vi "Modify Item.vi"(6 "Data":variant, 8 "error in (no error)":errorcluster, 9 "Text":string, 10 "Tag":refnum<class "Tree Tag Class.lvclass">, 11 "Tree_LVOOP in":refnum<class "Tree Class.lvclass">) -> (0 "error out":errorcluster, 2 "Tag dup":refnum<class "Tree Tag Class.lvclass">, 3 "Tree_LVOOP out":refnum<class "Tree Class.lvclass">)   [LabVIEW 2012, in "Tree Tools.lvlib" / "Tree Class.lvclass"]
uses:
  Tree Class.lvclass
  Tree Tag Class/Tree Tag Class.lvclass
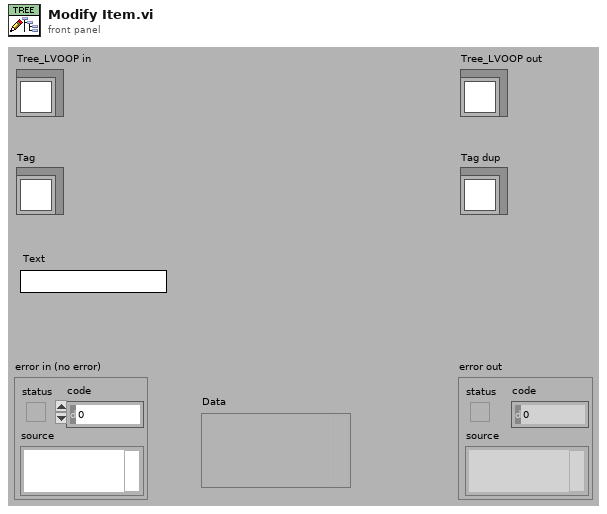
[diagram p1: front panel]
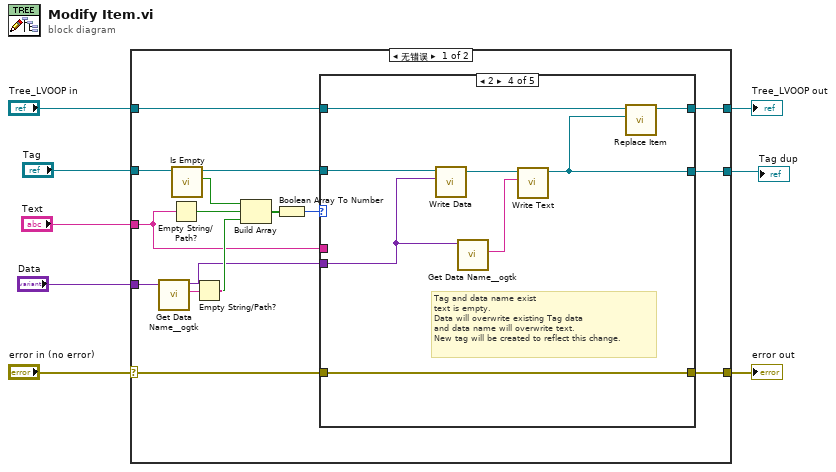
[diagram p0: block diagram]
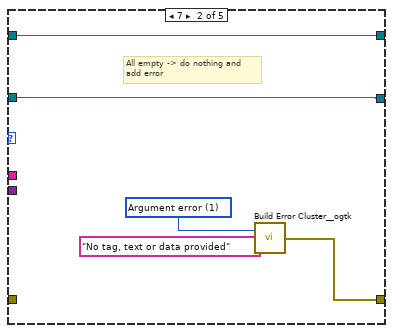
[diagram p3: hidden frame]
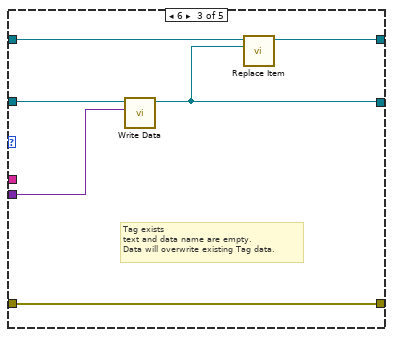
[diagram p4: hidden frame]
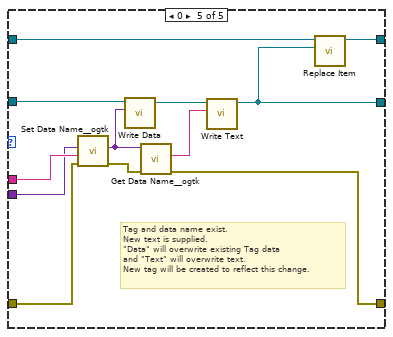
[diagram p5: hidden frame]
diagram:
  n1 = case shown="无错误" "error in (no error)" {
    selector: "error in (no error)" -> [w16 w61]
    tunnel: [w15 w61] -> w7
    tunnel: [w13 w60] -> w5
    tunnel: "Tree_LVOOP in" -> [w14 w60]
    tunnel: "Tag" -> [w24 w59]
    tunnel: "Text" -> [w11 _]
    tunnel: "Data" -> [w23 _]
    tunnel: [w9 w59] -> w1
    frame No Error {
      n2 = call <userlib>:"Get Data Name__ogtk.vi"("Data"=w23) -> ("Data Name"=w22:string, "Data dup"=w10:variant)  [unwired: 1 in, 8 out]
      n3 = Empty String/Path?(string/path=w11) -> (empty?=w20:bool)
      n4 = call-dynamic "Is Empty.vi"("Tag_LVOOP in"=w24) -> ("Empty"=w21:bool, "Tag_LVOOP out"=w12:refnum<class "Tree Tag Class.lvclass">)  [unwired: 8 in, 1 out]
      n5 = Empty String/Path?(string/path=w22) -> (empty?=w19:bool)
      n6 = Build Array(w21, w20, w19) -> (w18:bool[])
      n7 = Boolean Array To Number(Boolean array=w18) -> (number=w17:u32)
      n8 = case shown="2" w17 {
        tunnel: w16 -> [w26 _ w38 w46 w48]
        tunnel: [w26 w31 w38 w46 w47] -> w15
        tunnel: w14 -> [w27 w32 w35 w44 w57]
        tunnel: [w27 w32 w34 w43 w56] -> w13
        tunnel: w12 -> [w25 w28 w37 w45 w58]
        tunnel: w11 -> [_ _ _ _ w53]
        tunnel: w10 -> [_ _ w36 w41 w52]
        tunnel: [w25 w28 w33 w39 w54] -> w9
        frame Default {
        }
        frame 7 {
          w30 = 1 items=["No error", "Argument error", "Memory is full", "Out of zone", "End of file", "File already open", "Generic file I/O error", "File not found", "File permission error", "Disk is full", "Duplicate path", "Too many files open", "System feature not enabled", "Resource file not found", "Cannot add resource", "Resource not found", "Image not found", "Image memory error", "Pen does not exist", "Config type invalid", "Config token not found", "Config parse error", "Config memory error", "Bad external code format", "Bad external code offset", "External code not present", "Null window", "Destroy window error", "Null menu", "Print aborted", "Bad print record", "Print driver error", "Windows error during printing", "Memory error during printing", "Print dialog error", "Generic print error", "Invalid device refnum", "Device not found", "Device parameter error", "Device unit error", "Cannot open device", "Device call aborted", "Generic error", "Cancelled by user", "Object ID too low", "Object ID too high", "Object not in heap", "Unknown heap", "Unknown object (invalid DefProc)", "Unknown object (DefProc not in table)", "Message out of range", "Invalid (null) method", "Unknown message", "Manager call not supported", "Bad address", "Network operation in progress", "Network operation timed out", "Connection is busy", "Network attribute not supported", "Network error", "Address in use", "System out of memory", "Connection aborted", "Connection refused", "Not connected", "Already connected", "Connection closed", "Initialization error (interapplication manager)", "Bad occurrence", "Wait on unbound occurrence handler", "Occurrence queue overflow", "Datalog type conflict", "Unused", "Unrecognized type (interapplication manager)", "Memory corrupt", "Failed to make temporary DLL", "Old CIN version", "Drag socket not found", "Failed to load drop-object", "Failed to register OLE object", "Failed to release OLE object", "Format specifier type mismatch", "Unknown format specifier", "Too few format specifiers", "Too many format specifiers", "Scan failed", "Newer CIN version", "Error converting to variant", "Runtime menu error", "Password tampered", "Variant attribute not found", "Incompatible variant data type", "Event data is not available", "Event Store is not present", "Occurrence is not found", "Event Queue is not created", "Event info is not available", "Refnum passed is NULL", "Error retrieving Class GUID", "Error retrieving CoClass GUID", "Error retrieving TypeLib GUID.", "Bad built application magic bytes.", "Specific driver is different from the specific driver associated with the Logical Name.", "There is no session opened to the class driver.", "Max Error", "MAX - Error with config objects", "MAX - Error loading configuration", "MAX - Group not supported"]
          # "All empty -> do nothing and\nadd error"
          n9 = call <userlib>:"Build Error Cluster__ogtk.vi"("String to Prepend to source (\"\")"="No tag, text or data provided" ("String to Prepend to source (\"\")"), "code"=w30) -> ("error out"=w31:errorcluster)
        }
        frame 6 {
          # "Tag exists\ntext and data name are empty.\nData will overwrite existing Tag data."
          n10 = call-dynamic "Write Data.vi"("Data"=w36, "Tag_LVOOP.lvclass in"=w37) -> ("Tag_LVOOP.lvclass out"=w33:refnum<class "Tree Tag Class.lvclass">)  [unwired: 8 in, 1 out]
          n11 = call-dynamic "Replace Item.vi"("Tag"=w33, "Tree_LVOOP in"=w35) -> ("Tree_LVOOP out"=w34:refnum<class "Tree Class.lvclass">)  [unwired: 1 in, 8 out]
        }
        frame 2 {
          # "Tag and data name exist\ntext is empty.\nData will overwrite existing Tag data\nand data name will overwrite text.\nNew tag will be created to reflect this change."
          n12 = call-dynamic "Write Data.vi"("Data"=w41, "Tag_LVOOP.lvclass in"=w45) -> ("Tag_LVOOP.lvclass out"=w42:refnum<class "Tree Tag Class.lvclass">)  [unwired: 8 in, 1 out]
          n13 = call <userlib>:"Get Data Name__ogtk.vi"("Data"=w41) -> ("Data Name"=w40:string)  [unwired: 1 in, 9 out]
          n14 = call-dynamic "Write Text.vi"("Text"=w40, "Tag_LVOOP.lvclass in"=w42) -> ("Tag_LVOOP.lvclass out"=w39:refnum<class "Tree Tag Class.lvclass">)  [unwired: 8 in, 1 out]
          n15 = call-dynamic "Replace Item.vi"("Tag"=w39, "Tree_LVOOP in"=w44) -> ("Tree_LVOOP out"=w43:refnum<class "Tree Class.lvclass">)  [unwired: 1 in, 8 out]
        }
        frame 0 {
          # "Tag and data name exist.\nNew text is supplied.\n\"Data\" will overwrite existing Tag data\nand \"Text\" will overwrite text.\nNew tag will be created to reflect this change."
          n16 = call <userlib>:"Set Data Name__ogtk.vi"("error in (no error)"=w48, "Data Name"=w53, "Data"=w52) -> ("error out"=w49:errorcluster, "Renamed Data"=w51:variant)  [unwired: 7 out]
          n17 = call-dynamic "Write Data.vi"("Data"=w51, "Tag_LVOOP.lvclass in"=w58) -> ("Tag_LVOOP.lvclass out"=w55:refnum<class "Tree Tag Class.lvclass">)  [unwired: 8 in, 1 out]
          n18 = call <userlib>:"Get Data Name__ogtk.vi"("error in (no error)"=w49, "Data"=w51) -> ("error out"=w47:errorcluster, "Data Name"=w50:string)  [unwired: 8 out]
          n19 = call-dynamic "Write Text.vi"("Text"=w50, "Tag_LVOOP.lvclass in"=w55) -> ("Tag_LVOOP.lvclass out"=w54:refnum<class "Tree Tag Class.lvclass">)  [unwired: 8 in, 1 out]
          n20 = call-dynamic "Replace Item.vi"("Tag"=w54, "Tree_LVOOP in"=w57) -> ("Tree_LVOOP out"=w56:refnum<class "Tree Class.lvclass">)  [unwired: 1 in, 8 out]
        }
      }
    }
    frame Error {
    }
  }
  "error out" <- w7
  "Tree_LVOOP out" <- w5
  "Tag dup" <- w1
